vi "SensorReadOneLine1times.vi"(4 "EndPoint":T1 {"X" format="%#.5g"; "Y" format="%#.5g"; "Z" format="%#.6g"}, 6 "StartPoint":T1 {"X" format="%#.5g"; "Y" format="%#.5g"; "Z" format="%#.5g"}, 7 "file (use dialog)":path=path "C:/Users/TTUHEP/Documents/LabVIEW/output.txt", 8 "error out":errorcluster, 9 "Speed":dbl=2.0 format="%#_13g", 10 "VISA resource name":refnum<visa-resource-name>="COM4", 11 "controller":refnum<k24>) -> (0 "error out 2":errorcluster, 2 "VISA resource name out":refnum<visa-resource-name>, 3 "controller out":refnum<k24>)   [LabVIEW 2016]
uses:
  Control/Coordinate.ctl
  C:/Users/TTUHEP/Documents/LabVIEW/Other Models/2010/Bin/Aerotech.A3200.dll
  Other Models/2010/Bin/Aerotech.A3200.dll
  Other Models/2010/Status/ControllerDiagPacket.ctl
  Other Models/2010/Status/AxisDiagPacket.ctl
  <vilib>/Instr/_visa.llb/VISA Configure Serial Port (Instr).vi
panel:
  out "Boolean":bool=TRUE
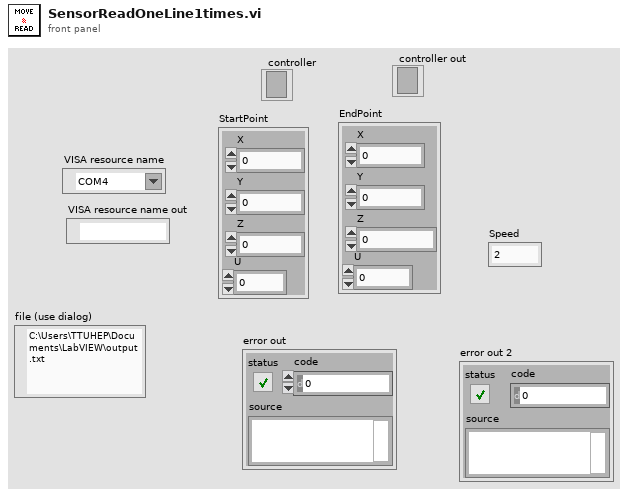
[diagram p1: front panel]
types:
  T1 = typedef "Coordinate.ctl" = cluster{"X":dbl, "Y":dbl, "Z":dbl, "U":dbl}
  T2 = typedef "ControllerDiagPacket.ctl" = cluster{"Number of Diag Packets":i32, "Axes":T3[], "error":errorcluster}
  T3 = typedef "AxisDiagPacket.ctl" = cluster{"Axis Name":string, "Analog Input 0":dbl, "Analog Input 1":dbl, "Axis Fault (num)":i32, "Axis Fault (str)":string, "Axis Fault (bits)":cluster{"AmplifierFault":bool, "AmplifierTemperatureFault":bool, "CcwEndOfTravelLimitFault":bool, "CcwSoftwareLimitFault":bool, "CommunicationLostFault":bool, "CwEndOfTravelLimitFault":bool, "CwSoftwareLimitFault":bool, "EmergencyStopFault":bool, "EncoderFault":bool, "ExternalFault":bool, "FeedbackScalingFault":bool, "GantryMisalignFault ":bool, "HallSensorFault":bool, "InPositionTimeoutFault":bool, "InternalFault":bool, "MarkerSearchFault":bool, "MaxVelocityCommandFault":bool, "MissedInterruptFault":bool, "MotorTemperatureFault":bool, "None":bool, "OverCurrentFault":bool, "PositionErrorFault":bool, "PositionFeedbackFault":bool, "PowerSupplyFault":bool, "ProbeInputFault":bool, "SafeZoneFault":bool, "VelocityErrorFault":bool, "VelocityFeedbackFault":bool, "VoltageClampFault":bool}, "Axis Status (num)":i32, "Axis Status (str)":string, "Axis Status (bits)":cluster{"BacklashActive":bool, "CalibrationEnabled1D":bool, "CalibrationEnabled2D":bool, "CommandValid":bool, "DriveAbortPending":bool, "DrivePending":bool, "Enabling":bool, "GainMappingEnabled":bool, "GantryAligned":bool, "GantryRealigning":bool, "Homed":bool, "Homing":bool, "IFOVEnabled":bool, "JogGenerating":bool, "Jogging":bool, "JoystickControl":bool, "MasterSlaveControl":bool, "MotionBlocked":bool, "MotionClamped":bool, "MoveDone":bool, "None":bool, "NotVirtual":bool, "Profiling":bool, "Stability0":bool, "Stability1":bool, "TrajectoryFiltering":bool, "WaitDone":bool}, "Current Command":sgl, "Current Error":sgl, "Current Feedback":sgl, "Digital Inputs":i32, "Digital Outputs":i32, "Drive Status":i32, "Drive Status (str)":string, "Drive Status (bits)":cluster{"AccelerationPhase":bool, "AutofocusActive":bool, "BrakeOutput":bool, "CcwEndOfTravelLimitInput":bool, "CosineEncoderError":bool, "CurrentClamp":bool, "CwEndOfTravelLimitInput":bool, "DecelerationPhase":bool, "DualLoopActive":bool, "EmergencyStopInput":bool, "Enabled":bool, "EncoderClipping":bool, "GalvoCalibrationEnabled":bool, "GalvoPowerCorrection":bool, "HallAInput":bool, "HallBInput":bool, "HallCInput":bool, "HighResolutionMode":bool, "HomeLimitInput":bool, "InPosition":bool, "InPosition2":bool, "MarkerInput":bool, "MarkerLatch":bool, "MoveActive":bool, "NoMotorSupply":bool, "None":bool, "PowerLimiting":bool, "ProgrammingFlash":bool, "ProgrammingMXH":bool, "PSOHaltLatch":bool, "ServoControl":bool, "SineEncoderError":bool}, "Position Feedback Auxiliary":dbl, "Position Command":dbl, "Position Error":dbl, "Position Feedback":dbl, "Program Position Command":dbl, "Program Position Error":dbl, "Program Position Feedback":dbl, "Velocity Command":dbl, "Velocity Error":dbl, "Velocity Feedback":dbl}
  T4 = cluster{"ControllerDiagPacket":T2, "read buffer":string}
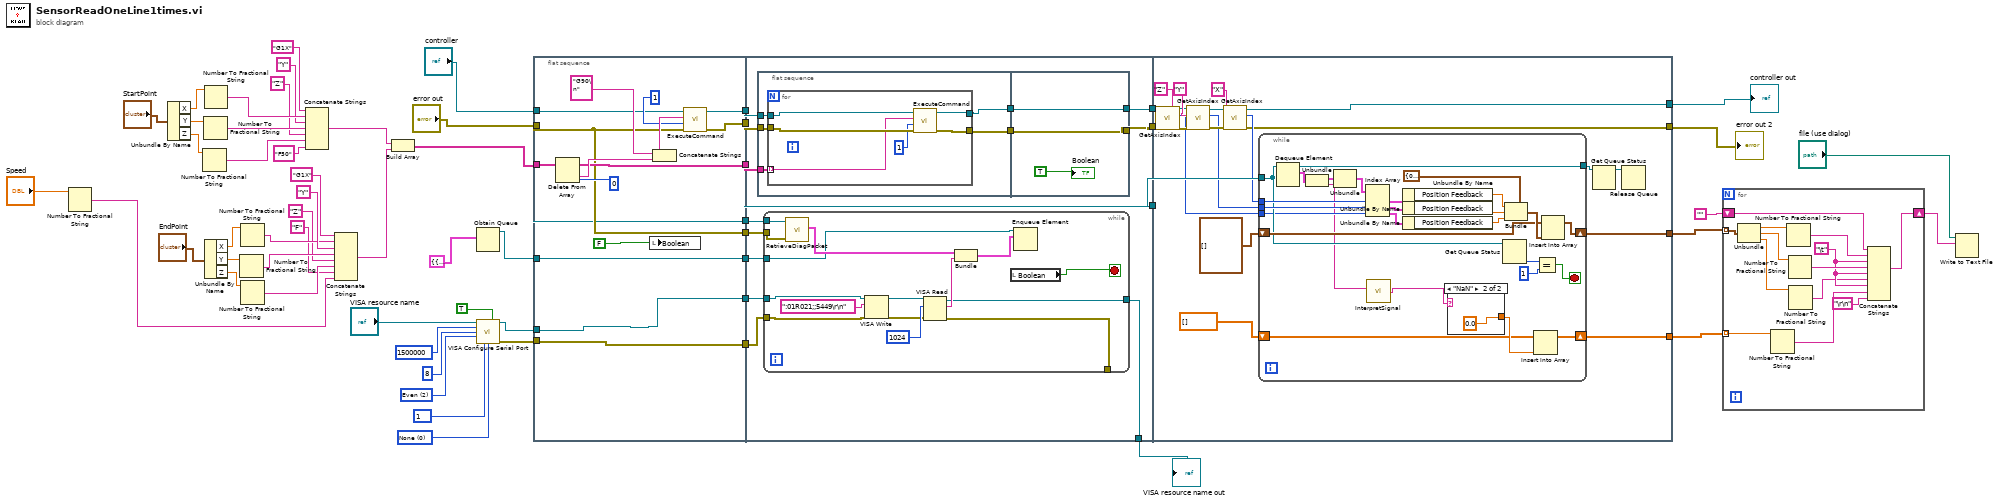
[diagram p0: block diagram]
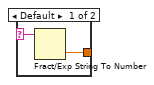
[diagram p2: hidden frame]
diagram:
  w9 = u16 0 items=["None"=0, "XON/XOFF"=1, "RTS/CTS"=2, "DTR/DSR"=4] ("flow control")
  w10 = u16 10 items=["1"=10, "1.5"=15, "2.0"=20] ("stop bits")
  w11 = u16 2 items=["None", "Odd", "Even", "Mark", "Space"] ("parity")
  n1 = Number To Fractional String(number="Speed") -> (F-format string=w16:string)  [unwired: 3 in]
  n2 = Unbundle By Name("StartPoint") -> ("X"=w47:dbl, "Y"=w46:dbl, "Z"=w22:dbl)
  n3 = Number To Fractional String(number=w22) -> (F-format string=w27:string)  [unwired: 3 in]
  n4 = Number To Fractional String(number=w46) -> (F-format string=w44:string)  [unwired: 3 in]
  n5 = Number To Fractional String(number=w47) -> (F-format string=w45:string)  [unwired: 3 in]
  n6 = Unbundle By Name("EndPoint") -> ("X"=w35:dbl, "Y"=w36:dbl, "Z"=w25:dbl)
  n7 = Number To Fractional String(number=w36) -> (F-format string=w38:string)  [unwired: 3 in]
  n8 = Number To Fractional String(number=w35) -> (F-format string=w37:string)  [unwired: 3 in]
  n9 = Number To Fractional String(number=w25) -> (F-format string=w24:string)  [unwired: 3 in]
  n10 = Concatenate Strings("G1X", w45, "Y", w44, "Z", w27, "F50") -> (w33:string)
  n11 = Concatenate Strings("G1X", w37, "Y", w38, "Z", w24, "F", w16) -> (w32:string)
  n12 = Build Array(w33, w32) -> (w31:string[])
  n13 = Obtain Queue(element data type=cluster{"ControllerDiagPacket":T2, string} {"ControllerDiagPacket"={"Number of Diag Packets"=0, "Axes"=[], "error"={"status"=FALSE, "code"=0, "source"=""}}, ""}) -> (queue out=w29:refnum<queue>)  [unwired: 4 in, 2 out]
  n14 = call-poly "VISA Configure Serial Port"("VISA resource name"="VISA resource name", "Enable Termination\nChar (T)"=TRUE, "baud rate (9600)"=u32 1500000 ("baud rate"), "data bits (8)"=u16 8 ("data bits"), "parity (0:none)"=w11, "stop bits (10: 1 bit)"=w10, "flow control (0:none)"=w9) -> ("VISA resource name out"=w6:refnum<visa-resource-name>, "error out"=w5:errorcluster)  [unwired: 7 in]
  n15 = flat-sequence {
    tunnel: [w68] -> w59
    tunnel: [w72] -> w58
    tunnel: [w73] -> w57
    tunnel: w31 -> [w74]
    tunnel: [w62] -> w56
    tunnel: [w63] -> w55
    tunnel: w29 -> [w66]
    tunnel: [w66] -> w54
    tunnel: [w61] -> w53
    tunnel: [w60] -> w52
    tunnel: "error out" -> [w63]
    tunnel: "controller" -> [w62]
    tunnel: w6 -> [w61]
    tunnel: w5 -> [w60]
    tunnel: [w82] -> w51
    tunnel: w59 -> [w76]
    tunnel: w58 -> [w78]
    tunnel: w57 -> [w77]
    tunnel: w56 -> [w86]
    tunnel: w55 -> [w87]
    tunnel: w54 -> [w85]
    tunnel: [w85] -> w50
    tunnel: w53 -> [w84]
    tunnel: w52 -> [w83]
    tunnel: [w79] -> w49
    tunnel: [w75] -> w2
    tunnel: w51 -> [w124]
    tunnel: w50 -> [w137]
    tunnel: [w126] -> w17
    tunnel: [w125] -> w18
    tunnel: w49 -> [w123]
    tunnel: [w118] -> w15
    tunnel: [w117] -> w14
    frame #0 {
      n16 = Delete From Array(array=w74, index=0) -> (deleted portion=w69:string, array with subset deleted=w68:string[])  [unwired: 1 in]
      n17 = local write "Boolean"(FALSE) -> ()
      n18 = Concatenate Strings("G90\n", w69) -> (w67:string)
      n19 = call "ExecuteCommand.vi"("error in (no error)"=w63, "taskId"=1, "Command Code"=w67, "controller in"=w62) -> ("error out"=w73:errorcluster, "controller out"=w72:refnum<k24>)  [unwired: 5 in, 1 out]
    }
    frame #1 {
      n20 = flat-sequence {
        tunnel: [w92] -> w81
        tunnel: [w91] -> w80
        tunnel: w78 -> [w90]
        tunnel: w77 -> [w89]
        tunnel: w76 -> [w88]
        tunnel: [w100] -> w82
        tunnel: w81 -> [w100]
        tunnel: w80 -> [w99]
        tunnel: [w99] -> w79
        frame #0 {
          n21 = for {
            tunnel: w88 -> [w96] mode=indexing
            tunnel: w90 -> [w97]
            tunnel: w89 -> [w98]
            tunnel: [w94] -> w92
            tunnel: [w93] -> w91
            n22 = call "ExecuteCommand.vi"("error in (no error)"=w98, "taskId"=1, "Command Code"=w96, "controller in"=w97) -> ("error out"=w94:errorcluster, "controller out"=w93:refnum<k24>)  [unwired: 5 in, 1 out]
          }
        }
        frame #1 {
          "Boolean" <- TRUE
        }
      }
      n23 = while {
        tunnel: w86 -> [w116]
        tunnel: w87 -> [w115]
        tunnel: w85 -> [w109]
        tunnel: w84 -> [w105]
        tunnel: w83 -> [w104]
        tunnel: [w108] -> w75
        tunnel: [w107] -> _
        stop <- w110 stop-if-true
        n24 = call "RetrieveDiagPacket.vi"("error in (no error)"=w115, "Controller In"=w116) -> ("ControllerDiagPacket"=w113:T2)  [unwired: 7 in, 2 out]
        n25 = VISA Write(VISA resource name=w105, write buffer=":01R021;;5449\r\n" ("Command"), error in (no error)=w104) -> (VISA resource name out=w102:refnum<visa-resource-name>, error out=w103:errorcluster)  [unwired: 1 out]
        n26 = VISA Read(VISA resource name=w102, byte count=u32 1024, error in (no error)=w103) -> (VISA resource name out=w108:refnum<visa-resource-name>, read buffer=w112:string, error out=w107:errorcluster)  [unwired: 1 out]
        n27 = Bundle("ControllerDiagPacket"=w113, "read buffer"=w112) -> (w111:T4)  [unwired: 1 in]
        n28 = local read "Boolean"() -> (w110:bool)
        n29 = Enqueue Element(queue=w109, element=w111) -> ()  [unwired: 2 in, 3 out]
      }
    }
    frame #2 {
      n30 = call "GetAxisIndex.vi"("error in (no error)"=w124, "axis name"="Z", "controller in"=w123) -> ("error out"=w121:errorcluster, "axis index"=w119:i32, "controller out"=w122:refnum<k24>)  [unwired: 6 in]
      n31 = call "GetAxisIndex.vi"("error in (no error)"=w121, "axis name"="Y", "controller in"=w122) -> ("error out"=w135:errorcluster, "axis index"=w131:i32, "controller out"=w136:refnum<k24>)  [unwired: 6 in]
      n32 = call "GetAxisIndex.vi"("error in (no error)"=w135, "axis name"="X", "controller in"=w136) -> ("error out"=w117:errorcluster, "axis index"=w132:i32, "controller out"=w118:refnum<k24>)  [unwired: 6 in]
      n33 = while {
        tunnel: w132 -> [w162]
        tunnel: w131 -> [w161]
        shift-right: [w154] -> w125
        shift-left: cluster{"X":dbl, "Y":dbl, "Y 2":dbl}[] [] -> [w152]
        tunnel: [w153] -> w129
        tunnel: w137 -> [w148]
        shift-right: [w143] -> w126
        shift-left: dbl[] [] -> [w144]
        tunnel: w119 -> [w142]
        stop <- w150 stop-if-true
        n34 = Dequeue Element(queue=w148) -> (queue out=w153:refnum<queue>, element=w147:cluster{"ControllerDiagPacket":T2, string})  [unwired: 2 in, 2 out]
        n35 = Unbundle(w147) -> ("ControllerDiagPacket"=w146:T2, w139:string)
        n36 = Unbundle(w146) -> ("Axes"=w163:T3[])  [unwired: 2 out]
        n37 = Index Array(array=w163, index #1=w162, index #2=w161, index #3=w142) -> (element #1=w160:T3, element #2=w159:T3, element #3=w141:T3)
        n38 = call "InterpretSignal.vi"("String in"=w139) -> ("String out"=w138:string)
        n39 = Unbundle By Name(w160) -> ("Position Feedback"=w157:dbl)
        n40 = Unbundle By Name(w159) -> ("Position Feedback"=w156:dbl)
        n41 = Unbundle By Name(w141) -> ("Position Feedback"=w140:dbl)
        n42 = case shown="\"NaN\"" w138 {
          selector: w138 -> [w165 _]
          tunnel: [w164 0.0] -> w145
          frame Default {
            n43 = Fract/Exp String To Number(string=w165) -> (number=w164:dbl)  [unwired: 3 in, 1 out]
          }
          frame "NaN" {
          }
        }
        n44 = Get Queue Status(queue=w148) -> (# elements in queue=w151:i32)  [unwired: 2 in, 7 out]
        n45 = Bundle(cluster=cluster{"X":dbl, "Y":dbl, "Z":dbl} {"X"=0.0, "Y"=0.0, "Z"=0.0}, "X"=w157, "Y"=w156, "Z"=w140) -> (w155:cluster{"X":dbl, "Y":dbl, "Z":dbl})
        n46 = Insert Into Array(array=w144, new element=w145) -> (w143:dbl[])  [unwired: 1 in]
        n47 = Equal?(x=w151, y=1) -> (x = y?=w150:bool)
        n48 = Insert Into Array(array=w152, new element=w155) -> (w154:cluster{"X":dbl, "Y":dbl, "Y 2":dbl}[])  [unwired: 1 in]
      }
      n49 = Get Queue Status(queue=w129) -> (queue out=w128:refnum<queue>)  [unwired: 2 in, 7 out]
      n50 = Release Queue(queue=w128) -> ()  [unwired: 2 in, 3 out]
    }
  }
  n51 = for {
    tunnel: w18 -> [w179] mode=indexing
    tunnel: w17 -> [w176] mode=indexing
    shift-right: [w172] -> w21
    shift-left: "" -> [w173]
    w171 = "\t"
    n52 = Unbundle(w179) -> ("X"=w178:dbl, "Y"=w177:dbl, "Y 2"=w170:dbl)
    n53 = Number To Fractional String(number=w176) -> (F-format string=w168:string)  [unwired: 3 in]
    n54 = Number To Fractional String(number=w178) -> (F-format string=w175:string)  [unwired: 3 in]
    n55 = Number To Fractional String(number=w177) -> (F-format string=w174:string)  [unwired: 3 in]
    n56 = Number To Fractional String(number=w170) -> (F-format string=w169:string)  [unwired: 3 in]
    n57 = Concatenate Strings(w173, w175, w171, w174, w171, w169, w171, w168, "\r\n") -> (w172:string)
  }
  n58 = Write to Text File(file (use dialog)="file (use dialog)", text=w21) -> ()  [unwired: 2 in, 3 out]
  "controller out" <- w15
  "error out 2" <- w14
  "VISA resource name out" <- w2
